vi "tt1.vi"   [LabVIEW 2010]
uses:
  全局量/全局_配置.vi
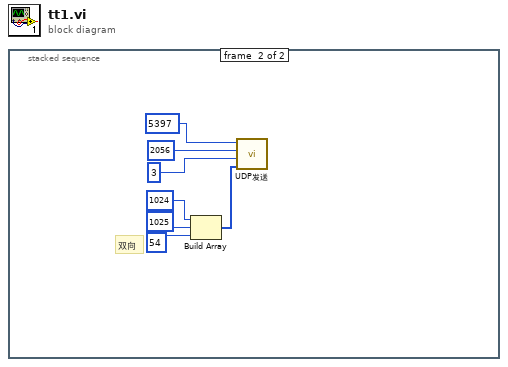
[diagram p0: block diagram]
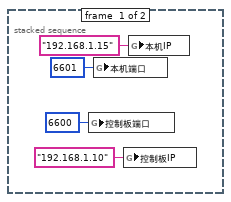
[diagram p2: hidden frame]
diagram:
  n1 = stacked-sequence {
    frame #0 {
      n2 = global write "全局_配置.vi" "控制板端口"(u16 6600 ("控制板端口")) -> ()
      n3 = global write "全局_配置.vi" "本机端口"(u16 6601 ("本机端口")) -> ()
      n4 = global write "全局_配置.vi" "控制板IP"("192.168.1.10" ("控制板IP")) -> ()
      n5 = global write "全局_配置.vi" "本机IP"("192.168.1.15" ("本机IP")) -> ()
    }
    frame #1 {
      # "双向"
      n6 = Build Array(u16 1024, u16 1025, u16 54) -> (w5:u16[])
      n7 = call "UDP发送.vi"("发送数据"=w5, "数据区字长"=u16 3, "报文类型"=u16 2056, "发送方标识"=u16 5397) -> ()  [unwired: 7 in]
    }
  }
